vi "Write_AddProcess.vi"(8 "error in (no error)":errorcluster, 10 "Process in":refnum<class "Process.lvclass">, 11 "EVE.lvclass in":refnum<class "EVE.lvclass">) -> (0 "error out":errorcluster, 3 "EVE.lvclass out":refnum<class "EVE.lvclass">)   [LabVIEW 2013, in "EVE.lvclass"]
uses:
  EVE.lvclass
  100_PROCESS/Class/Process/Process.lvclass
  EVE.lvclass/EVE.ctl
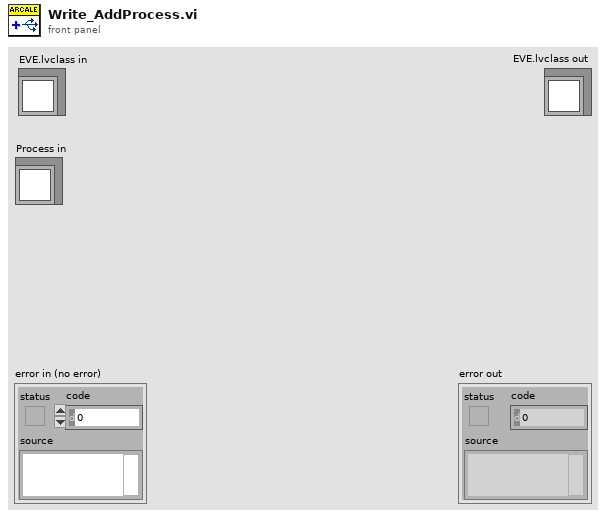
[diagram p1: front panel]
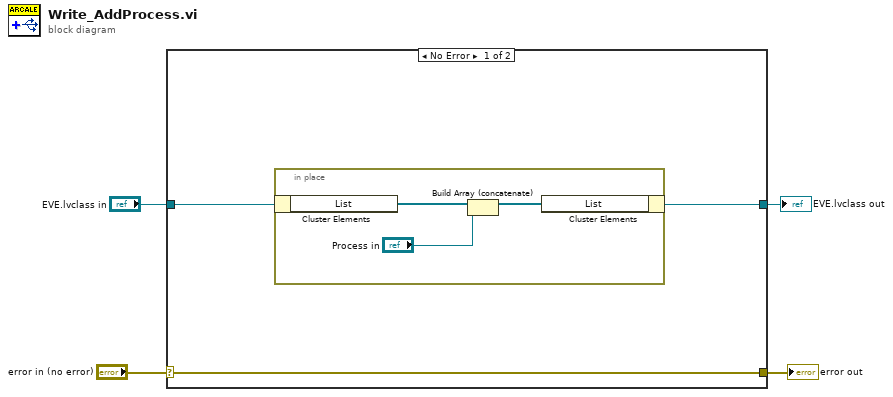
[diagram p0: block diagram]
diagram:
  n1 = case shown="No Error" "error in (no error)" {
    selector: "error in (no error)" -> [w7 w12]
    tunnel: [w7 w12] -> w3
    tunnel: [w5 w11] -> w1
    tunnel: "EVE.lvclass in" -> [w6 w11]
    frame No Error {
      n2 = in-place {
        n3 = in-place-cluster #1(w6) -> ("List"=w10:refnum<class "Process.lvclass">[])
        n4 = Build Array (concatenate)(w10, "Process in") -> (w8:refnum<class "Process.lvclass">[])
        n5 = in-place-cluster #1("List"=w8) -> (w5:refnum<class "EVE.lvclass">)
      }
    }
    frame Error {
    }
  }
  "error out" <- w3
  "EVE.lvclass out" <- w1
